vi "Initialize.vi"(8 "error in":errorcluster, 11 "Plugin in":refnum<class "StreamWriter.lvclass">) -> (0 "error out":errorcluster, 3 "Plugin out":refnum<class "StreamWriter.lvclass">)   [LabVIEW 2024, in "StreamWriter.lvlib" / "StreamWriter.lvclass"]
uses:
  StreamWriter.lvclass
  C:/Program Files/National Instruments/LabVIEW 2024/vi.lib/FlexLogger/SDK/PluginSDK.lvlibp/PEFClasses/SDK/Plugin/Plugin.lvclass
  <vilib>/FlexLogger/SDK/PluginSDK.lvlibp/PEFClasses/SDK/Processing Element/Timing Parameters.ctl
  <vilib>/FlexLogger/SDK/PluginSDK.lvlibp/PEFClasses/SDK/Processing Element/Timing Method.ctl
  StreamWriter Strings.vi
  <vilib>/FlexLogger/SDK/PluginSDK.lvlibp/PEFClasses/SDK/Plugin/ParameterAccess/Write String.vi
  <vilib>/FlexLogger/SDK/PluginSDK.lvlibp/PEFClasses/SDK/Plugin/ParameterAccess/Write I32.vi
  <vilib>/FlexLogger/SDK/PluginSDK.lvlibp/PEFClasses/SDK/Plugin/ParameterAccess/Write N Channel.vi
  <vilib>/FlexLogger/SDK/PluginSDK.lvlibp/PEFClasses/SDK/Plugin/Plugin.lvclass
  <vilib>/FlexLogger/SDK/PluginSDK.lvlibp/PEFClasses/SDK/Processing Element/Processing Element.lvclass
  C:/Program Files/National Instruments/LabVIEW 2024/vi.lib/FlexLogger/SDK/PluginSDK.lvlibp/PEFClasses/SDK/Processing Element/Processing Element.lvclass
  C:/dev/niflexlogger-plugins/plugins/StreamWriter/source/StreamWriter.lvclass
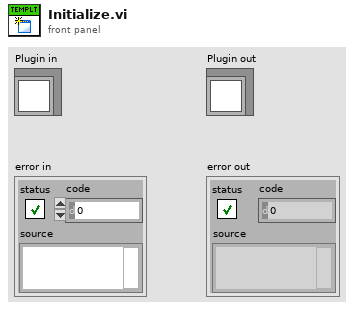
[diagram p1: front panel]
types:
  T1 = typedef "PluginSDK.lvlibp/Processing Element.lvclass/Timing Parameters.ctl" = cluster{"Timing Method":T2, "Timing Period (ms)":i32}
  T2 = typedef "PluginSDK.lvlibp/Processing Element.lvclass/Timing Method.ctl" = enum16{"Periodic", "Immediate", "On Data Ready", "Triggered"}
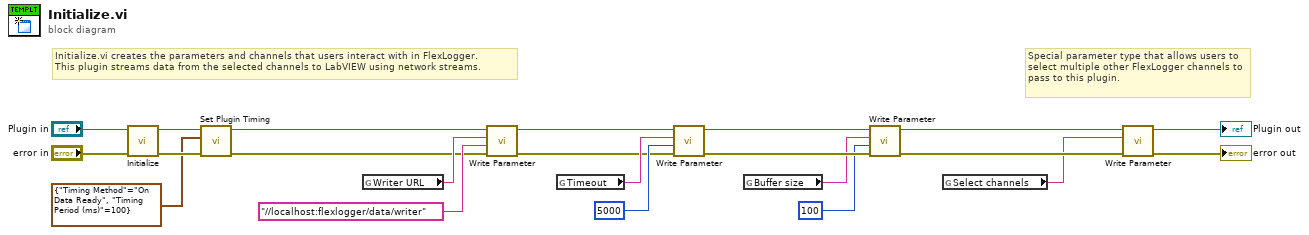
[diagram p0: block diagram]
diagram:
  # "Special parameter type that allows users to select multiple other FlexLogger channels to pass to this plugin."
  # "Initialize.vi creates the parameters and channels that users interact with in FlexLogger.\nThis plugin streams data from the selected channels to LabVIEW using network streams."
  n1 = call-parent "Initialize.vi"("error in (no error)"="error in", "Plugin in"="Plugin in") -> ("error out"=w21:errorcluster, "Plugin out"=w22:refnum<class "StreamWriter.lvclass">)  [unwired: 8 in]
  n2 = call <vilib>:"Set Plugin Timing.vi"("error in (no error)"=w21, "Timing Parameters"=T1 {"Timing Method"=enum."On Data Ready", "Timing Period (ms)"=100}, "Plugin in"=w22) -> ("error out"=w3:errorcluster, "Plugin out"=w4:refnum<class "StreamWriter.lvclass">)  [unwired: 7 in]
  n3 = global read "StreamWriter Strings.vi" "Writer URL"() -> (w6:string)
  n4 = call-poly <vilib>:"Write Parameter.vi"("error in (no error)"=w3, "Value"="//localhost:flexlogger/data/writer", "Name"=w6, "Plugin in"=w4) -> ("error out"=w2:errorcluster, "Plugin out"=w1:refnum<class "StreamWriter.lvclass">)  [unwired: 6 in]
  n5 = global read "StreamWriter Strings.vi" "Timeout"() -> (w9:string)
  n6 = call-poly <vilib>:"Write Parameter.vi"("error in (no error)"=w2, "Value"=5000, "Name"=w9, "Plugin in"=w1) -> ("error out"=w17:errorcluster, "Plugin out"=w19:refnum<class "StreamWriter.lvclass">)  [unwired: 6 in]
  n7 = global read "StreamWriter Strings.vi" "Buffer size"() -> (w8:string)
  n8 = call-poly <vilib>:"Write Parameter.vi"("error in (no error)"=w17, "Value"=100, "Name"=w8, "Plugin in"=w19) -> ("error out"=w16:errorcluster, "Plugin out"=w18:refnum<class "StreamWriter.lvclass">)  [unwired: 6 in]
  n9 = global read "StreamWriter Strings.vi" "Select channels"() -> (w7:string)
  n10 = call-poly <vilib>:"Write Parameter.vi"("error in (no error)"=w16, "Name (Unique Channel Identifier)"=w7, "Plugin in"=w18) -> ("error out"=→"error out":errorcluster, "Plugin out"=→"Plugin out":refnum<class "StreamWriter.lvclass">)  [unwired: 7 in]
